vi "Function Generator.vi"() -> ()   [LabVIEW 2016]
uses:
  QSM-PC (String)/Library/QSM-PC (String).lvlib
  <vilib>/measure/NI_MABase.lvlib
panel:
  out "波形图表":waveform(dbl)(graph)
  out "QSM - Function_Generator":refnum<queue>
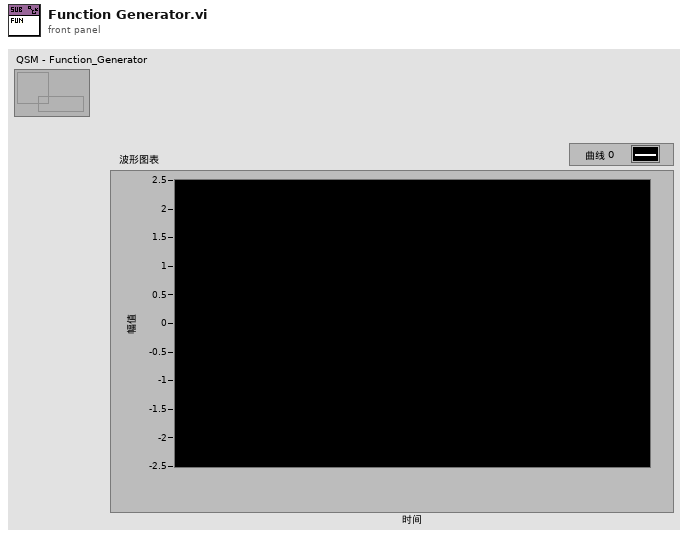
[diagram p1: front panel]
types:
  T1 = cluster{"DevType":string, "DevName":string, "Function":cluster{"signaltype":string, "frequency":dbl, "amplitude":dbl, "phase":dbl}[]}
  T2 = cluster{"signaltype":string, "frequency":dbl, "amplitude":dbl, "phase":dbl}[]
  T3 = cluster{"signaltype":string, "frequency":dbl, "amplitude":dbl, "phase":dbl}
  T4 = enum16{"Sine Wave", "Triangle Wave", "Square Wave", "Sawtooth Wave"}
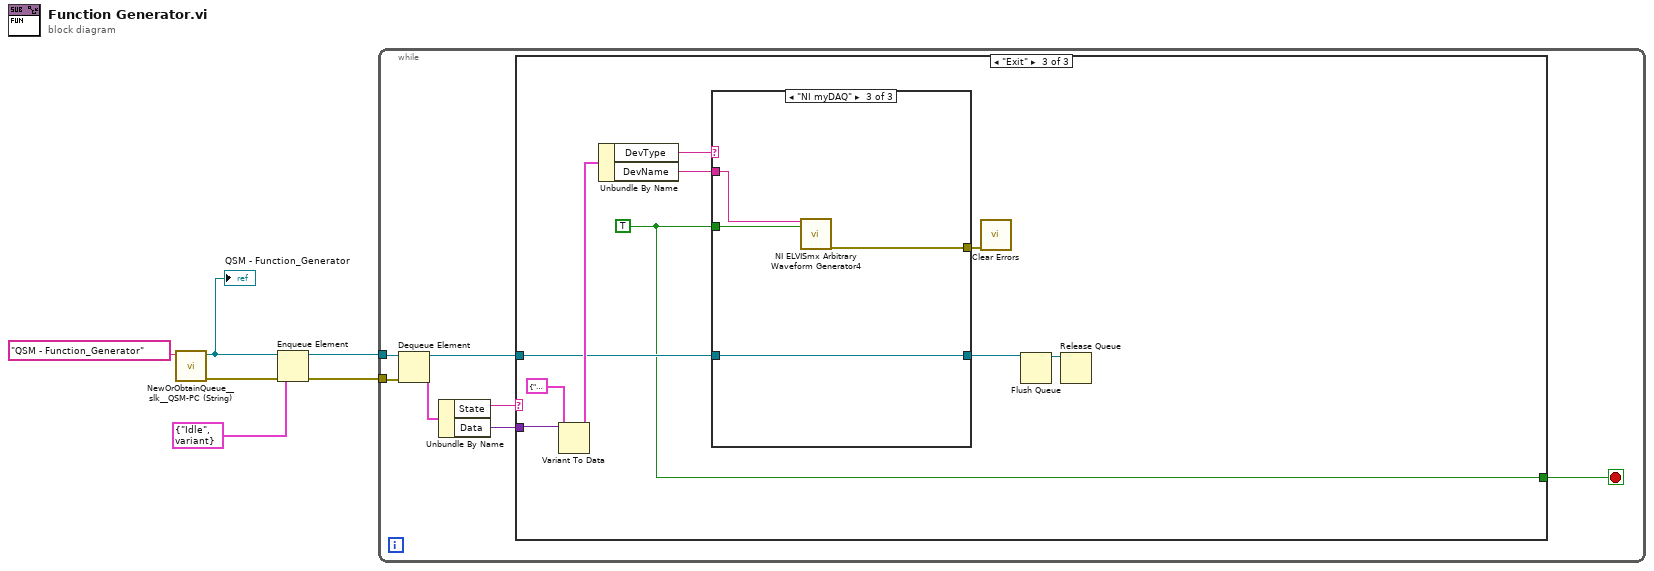
[diagram p0: block diagram]
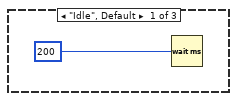
[diagram p2: hidden frame]
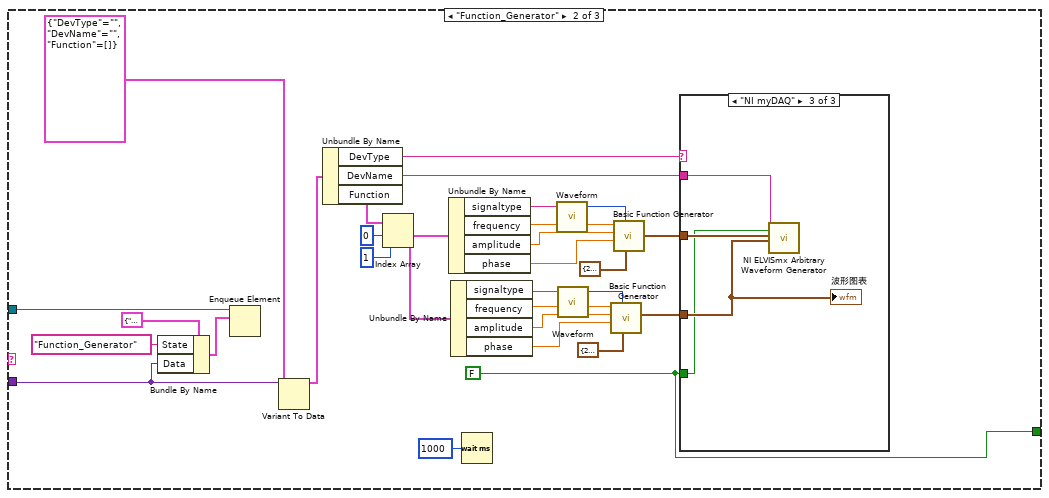
[diagram p3: hidden frame]
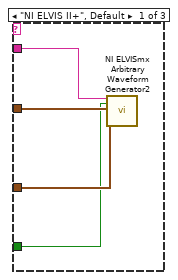
[diagram p4: hidden frame]
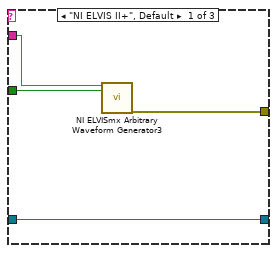
[diagram p6: hidden frame]
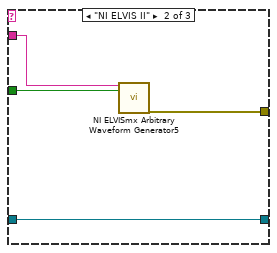
[diagram p7: hidden frame]
diagram:
  n1 = call "NewOrObtainQueue__slk__QSM-PC (String).vi"("queue name in"="QSM - Function_Generator") -> ("error out"=w5:errorcluster, "queue out"=w6:refnum<queue>)  [unwired: 2 in, 7 out]
  "QSM - Function_Generator" <- w6
  n2 = Enqueue Element(queue=w6, element=cluster{"State":string, "Data":variant} {"State"="Idle", "Data"=variant} ("元素"), error in (no error)=w5) -> (queue out=w2:refnum<queue>, error out=w1:errorcluster)  [unwired: 2 out]
  n3 = while {
    tunnel: w2 -> [w13]
    tunnel: w1 -> [w12]
    stop <- w7 stop-if-true
    n4 = Dequeue Element(queue=w13, error in (no error)=w12) -> (queue out=w10:refnum<queue>, element=w11:cluster{"State":string, "Data":variant})  [unwired: 1 in, 2 out]
    n5 = Unbundle By Name(w11) -> ("State"=w9:string, "Data"=w8:variant)
    n6 = case shown="\"Exit\"" w9 {
      tunnel: w10 -> [_ w23 w56]
      tunnel: w8 -> [_ w16 w60]
      tunnel: [_ w15 w54] -> w7
      frame "Idle", Default {
        n7 = Wait (ms)(milliseconds to wait=u32 200 ("等待时间（毫秒）")) -> ()  [unwired: 1 out]
      }
      frame "Function_Generator" {
        w15 = FALSE
        n8 = Bundle By Name(cluster=cluster{"State":string, "Data":variant} {"State"="", "Data"=variant} ("元素"), "State"="Function_Generator", "Data"=w16) -> (w21:cluster{"State":string, "Data":variant})
        n9 = Enqueue Element(queue=w23, element=w21) -> ()  [unwired: 2 in, 3 out]
        n10 = Variant To Data(type=T1 {"DevType"="", "DevName"="", "Function"=[]}, Variant=w16) -> (data=w17:T1)  [unwired: 1 in, 1 out]
        n11 = Unbundle By Name(w17) -> ("DevType"=w43:string, "DevName"=w42:string, "Function"=w39:T2)
        n12 = Index Array(array=w39, index #1=0 ("索引"), index #2=1 ("索引")) -> (element #1=w38:T3, element #2=w34:T3)
        n13 = Unbundle By Name(w38) -> ("signaltype"=w28:string, "frequency"=w37:dbl, "amplitude"=w36:dbl, "phase"=w35:dbl)
        n14 = Unbundle By Name(w34) -> ("signaltype"=w26:string, "frequency"=w31:dbl, "amplitude"=w30:dbl, "phase"=w29:dbl)
        n15 = Wait (ms)(milliseconds to wait=u32 1000 ("等待时间（毫秒）")) -> ()  [unwired: 1 out]
        n16 = call "Waveform.vi"("signal type"=w28) -> ("signal type"=w27:T4)  [unwired: 4 in]
        n17 = call "Waveform.vi"("signal type"=w26) -> ("signal type"=w25:T4)  [unwired: 4 in]
        n18 = call <vilib>:"Basic Function Generator.vi"("sampling info"=cluster{"Fs":dbl, "#s":dbl} {"Fs"=200000.0, "#s"=200000.0}, "signal type"=w25, "phase"=w29, "amplitude"=w30, "frequency"=w31) -> ("signal out"=w40:waveform(dbl))  [unwired: 4 in, 2 out]
        n19 = call <vilib>:"Basic Function Generator.vi"("sampling info"=cluster{"Fs":dbl, "#s":dbl} {"Fs"=200000.0, "#s"=200000.0}, "signal type"=w27, "phase"=w35, "amplitude"=w36, "frequency"=w37) -> ("signal out"=w41:waveform(dbl))  [unwired: 4 in, 2 out]
        n20 = case shown="\"NI myDAQ\"" w43 {
          tunnel: w42 -> [w48 _ w52]
          tunnel: w41 -> [w47 _ w51]
          tunnel: w40 -> [w46 _ w50]
          tunnel: w15 -> [w45 _ w49]
          frame "NI ELVIS II+", Default {
            n21 = call "NI ELVISmx Arbitrary Waveform Generator2"("Device Name"=w48, "Stop"=w45, "Channel 0 Signal In"=w47, "Channel 1 Signal In"=w46) -> ()  [unwired: 15 in, 1 out]
          }
          frame "NI ELVIS II" {
          }
          frame "NI myDAQ" {
            n22 = call "NI ELVISmx Arbitrary Waveform Generator"("Device Name"=w52, "Stop"=w49, "Channel 0 Signal In"=w51, "Channel 1 Signal In"=w50) -> ()  [unwired: 15 in, 1 out]
            "波形图表" <- w50
          }
        }
      }
      frame "Exit" {
        w54 = TRUE
        n23 = Variant To Data(type=T1 {"DevType"="", "DevName"="", "Function"=[]}, Variant=w60) -> (data=w59:T1)  [unwired: 1 in, 1 out]
        n24 = Unbundle By Name(w59) -> ("DevType"=w58:string, "DevName"=w57:string)
        n25 = case shown="\"NI myDAQ\"" w58 {
          tunnel: w57 -> [w66 w68 w74]
          tunnel: w54 -> [w65 w67 w73]
          tunnel: w56 -> [w64 w70 w72]
          tunnel: [w64 w70 w72] -> w55
          tunnel: [w63 w69 w71] -> w53
          frame "NI ELVIS II+", Default {
            n26 = call "NI ELVISmx Arbitrary Waveform Generator3"("Device Name"=w66, "Stop"=w65) -> ("error out"=w63:errorcluster)  [unwired: 17 in]
          }
          frame "NI ELVIS II" {
            n27 = call "NI ELVISmx Arbitrary Waveform Generator5"("Device Name"=w68, "Stop"=w67) -> ("error out"=w69:errorcluster)  [unwired: 17 in]
          }
          frame "NI myDAQ" {
            n28 = call "NI ELVISmx Arbitrary Waveform Generator4"("Device Name"=w74, "Stop"=w73) -> ("error out"=w71:errorcluster)  [unwired: 17 in]
          }
        }
        n29 = call <vilib>:"Clear Errors.vi"("error in (no error)"=w53) -> ()  [unwired: 5 in, 2 out]
        n30 = Flush Queue(queue=w55) -> (queue out=w62:refnum<queue>)  [unwired: 1 in, 2 out]
        n31 = Release Queue(queue=w62) -> ()  [unwired: 2 in, 3 out]
      }
    }
  }
